vi "Initialize FIFOs.vi"(8 "error in (no error)":errorcluster, 10 "Data Access":refnum<class "Data Access Engine.lvclass">, 11 "Channel Reader in":refnum<class "Channel Manager.lvclass">) -> (0 "error out":errorcluster, 3 "Channel Reader out":refnum<class "Channel Manager.lvclass">)   [LabVIEW 2024, in "Embedded TDMS Logger Engine.lvlib" / "Channel Manager.lvclass"]
doc: "Get references to the data access engine FIFO's it has setup for our CD channels which are managed by the RT Driver VI and communicates asynchronously with the VeriStand Engine."
uses:
  Channel Manager.lvclass
  <vilib>/NI/NIVS Inline Async API/_Data Access Engine/Data Access Engine/Data Access Engine.lvclass
  Channel Manager.lvclass/Channel Manager.ctl
  <vilib>/NI/NIVS Inline Async API/_Data Access Engine/Data Access Engine/Methods/Read.Lookup.vi
  <vilib>/NI/NIVS Inline Async API/_Data Access Engine/Data Access Engine/Methods/Write.Lookup.vi
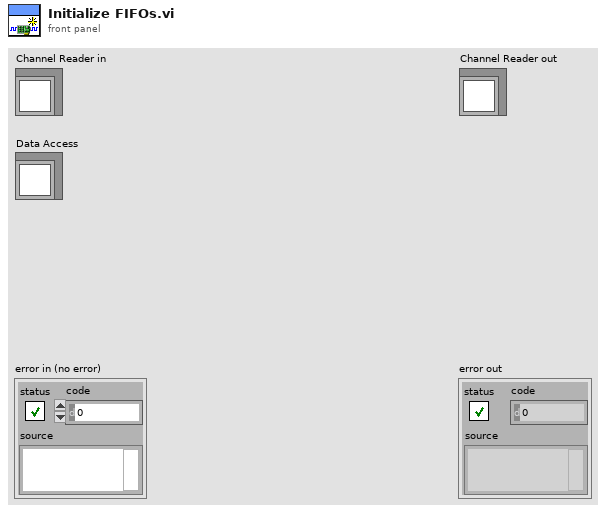
[diagram p1: front panel]
types:
  T1 = typedef "Data Access Engine.lvlib/Data Access Engine.lvclass/Read.DVR.ctl" = refnum<data-value>
  T2 = typedef "Data Access Engine.lvlib/Data Access Engine.lvclass/Write.DVR.ctl" = refnum<data-value>
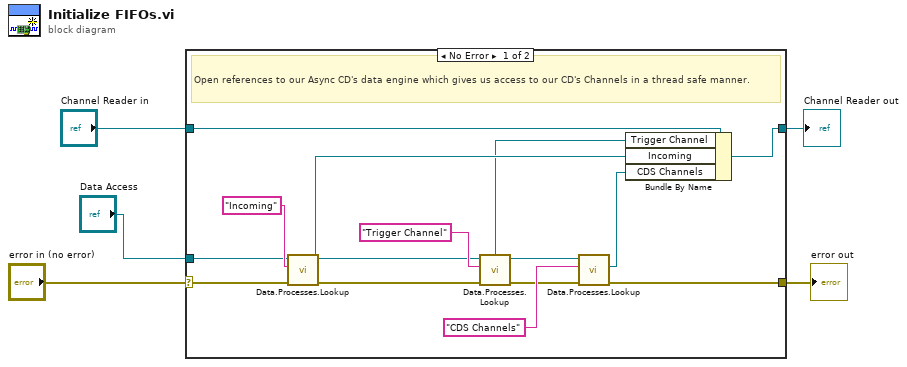
[diagram p0: block diagram]
diagram:
  n1 = case shown="No Error" "error in (no error)" {
    selector: "error in (no error)" -> [w13 w22]
    tunnel: [w12 w22] -> w4
    tunnel: [w10 w21] -> w2
    tunnel: "Channel Reader in" -> [w11 w21]
    tunnel: "Data Access" -> [w6 _]
    frame No Error {
      # "Open references to our Async CD's data engine which gives us access to our CD's Channels in a thread safe manner."
      n2 = call-poly <vilib>:"Data.Processes.Lookup.vi"("error in (no error)"=w13, "Name"="Incoming", "Data Access API in"=w6) -> ("error out"=w18:errorcluster, "Ref"=w8:T1, "Data Access API out"=w17:refnum<class "Data Access Engine.lvclass">)  [unwired: 5 in, 1 out]
      n3 = call-poly <vilib>:"Data.Processes.Lookup.vi"("error in (no error)"=w18, "Name"="Trigger Channel", "Data Access API in"=w17) -> ("error out"=w15:errorcluster, "Ref"=w7:T1, "Data Access API out"=w14:refnum<class "Data Access Engine.lvclass">)  [unwired: 5 in, 1 out]
      n4 = call-poly <vilib>:"Data.Processes.Lookup.vi"("error in (no error)"=w15, "Name"="CDS Channels", "Data Access API in"=w14) -> ("error out"=w12:errorcluster, "Ref"=w9:T2)  [unwired: 5 in, 2 out]
      n5 = Bundle By Name(cluster=w11, "Trigger Channel"=w7, "Incoming"=w8, "CDS Channels"=w9) -> (w10:refnum<class "Channel Manager.lvclass">)
    }
    frame Error {
    }
  }
  "error out" <- w4
  "Channel Reader out" <- w2
